vi "Test2_3b.vi"(0 "Instrument VISA in":T1={"AWG VISA"="81160A", "Oscilloscope  VISA "="Oscilloscope", "Integration Board IP"="172.16.7.43", "connection ID"=refnum, "report out"=refnum, "report file path"=path "D:/CTA/Data_test/adds"}, 7 "Cycles Burst":i32=10000, 9 "L1 Address":i32=17, 11 "error in":errorcluster, 12 "channel array":i32[](array[numeric])=[0, 1, 2, 3, 4, 5, 6], 13 "L1 version":bool) -> (4 "Instrument VISA out":T1={"AWG VISA"="81160A", "Oscilloscope  VISA "="Oscilloscope", "Integration Board IP"="172.16.7.43", "connection ID"=refnum, "report out"=refnum, "report file path"=path "D:/CTA/Data_test/adds"}, 15 "error out":errorcluster)   [LabVIEW 2009]
uses:
  <vilib>/Utility/NIReport.llb/NI_report.lvclass
  <instrlib>/Agilent 81150/Agilent 81150.lvlib
  <instrlib>/Agilent 8000 Series/Agilent 8000 Series.lvlib
panel:
  in  "Voltage":dbl[](array[numeric])=[0.05, 0.1, 0.2, 0.3, 0.4, 0.5, 0.6, 0.7, 0.8, 0.9, 1.0, 1.1, 1.2]
  in  "quantity":i32=2
  in  "cliipping":i32[](array[numeric])=[380, 381, 396, 376, 369, 371, 333]
  in  "attenuation":i32[](array[numeric])=[1574, 1572, 1542, 1574, 1569, 1563, 1581]
  out "IPR_Address":i32=23
  out "L1 Address":i32=17
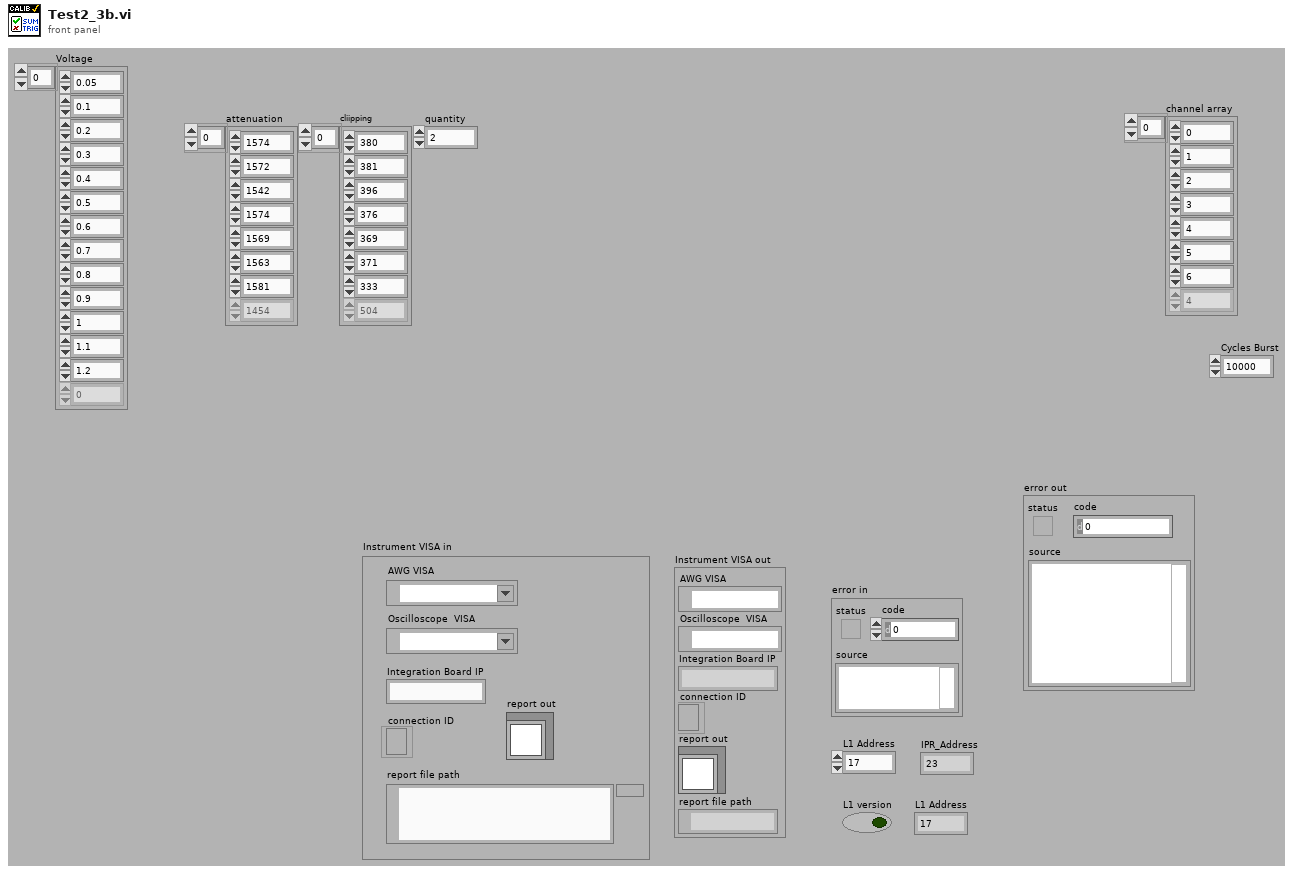
[diagram p1: front panel]
types:
  T1 = cluster{"AWG VISA":refnum<visa-resource-name>, "Oscilloscope  VISA ":refnum<visa-resource-name>, "Integration Board IP":string, "connection ID":refnum<k5>, "report out":refnum<class "NI_report.lvclass">, "report file path":path}
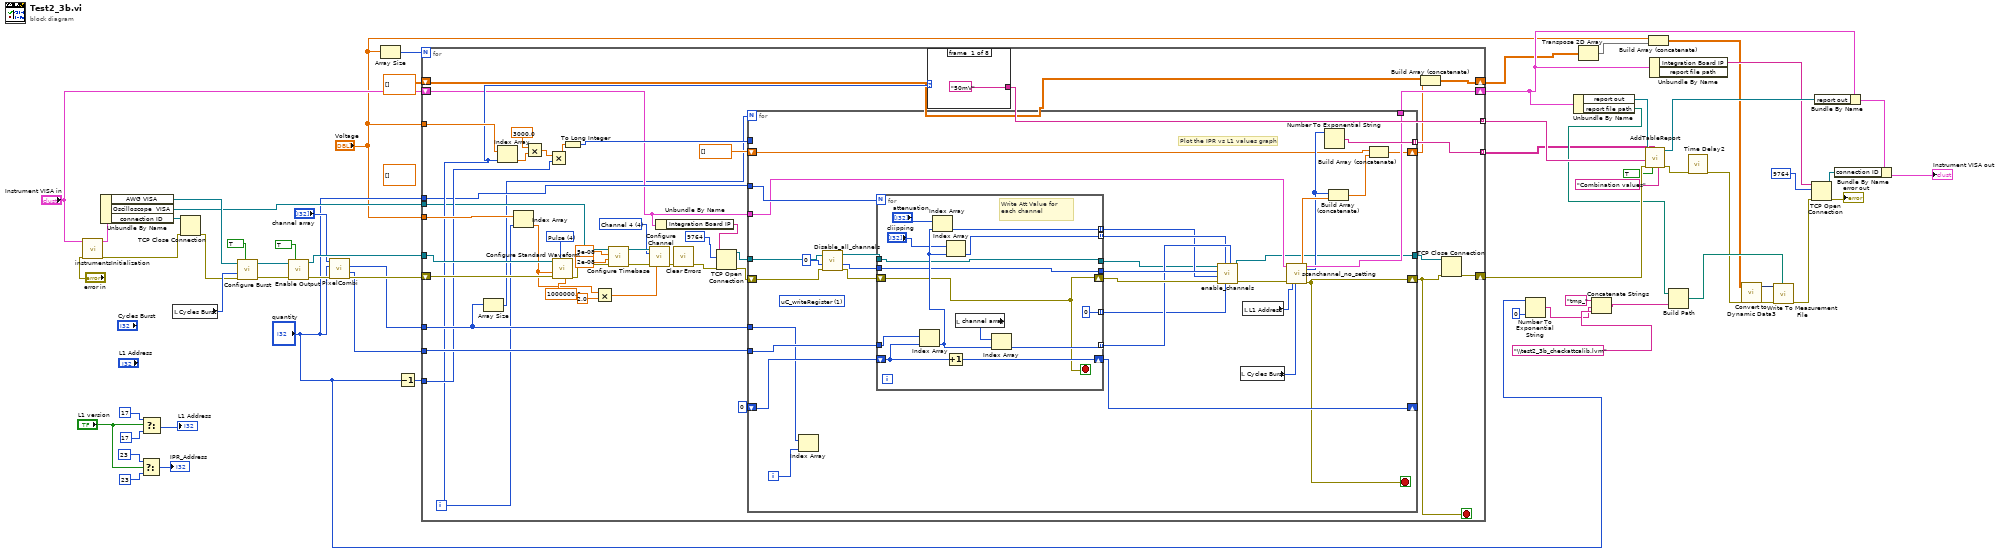
[diagram p0: block diagram]
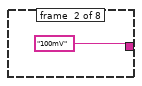
[diagram p2: hidden frame]
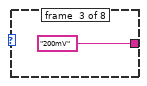
[diagram p3: hidden frame]
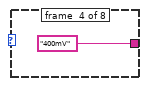
[diagram p4: hidden frame]
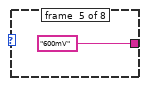
[diagram p5: hidden frame]
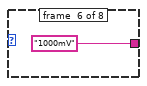
[diagram p6: hidden frame]
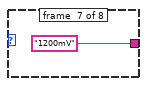
[diagram p7: hidden frame]
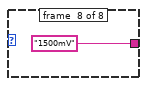
[diagram p8: hidden frame]
diagram:
  (unwired) dbl[][] []
  n1 = call "instrumentsInitialization.vi"("error in"="error in", "Instrument VISA in"="Instrument VISA in") -> ("error out"=w18:errorcluster, "Instrument VISA out"=w20:T1)  [unwired: 8 in]
  n2 = Unbundle By Name(w20) -> ("AWG VISA"=w21:refnum<visa-resource-name>, "Oscilloscope  VISA"=w16:refnum<visa-resource-name>, "connection ID"=w19:refnum<k5>)
  n3 = Select(t=23 ("Address"), s="L1 version", f=23 ("Address")) -> (s? t:f=→"IPR_Address":i32)
  n4 = Select(t=17 ("Address"), s="L1 version", f=17 ("Address")) -> (s? t:f=→"L1 Address":i32)
  n5 = local read "Cycles Burst"() -> (w57:i32)
  n6 = TCP Close Connection(connection ID=w19, error in (no error)=w18) -> (error out=w17:errorcluster)  [unwired: 1 in, 1 out]
  n7 = call <instrlib>:"Configure Burst.vi"("Enable Burst (F: Disable)"=TRUE, "error in (no error)"=w17, "Burst Count (2)"=w57, "VISA resource name"=w21) -> ("error out"=w56:errorcluster, "VISA resource name out"=w55:refnum<visa-resource-name>)  [unwired: 6 in]
  n8 = call <instrlib>:"Enable Output.vi"("Enable Output (T: Enable)"=TRUE, "error in (no error)"=w56, "VISA resource name"=w55) -> ("error out"=w54:errorcluster, "VISA resource name out"=w52:refnum<visa-resource-name>)  [unwired: 7 in]
  n9 = call "PixelCombi.vi"("error in"=w54, "quantity"="quantity", "array"="channel array") -> ("error out"=w53:errorcluster, "Channels"=w51:i32[], "Combination Array"=w50:i16[])  [unwired: 6 in]
  n10 = Array Size(array="Voltage") -> (size(s)=w24:i32)
  n11 = Decrement(x="quantity") -> (x-1=w23:i32)
  n12 = for {
    N: w24 -> [_]
    tunnel: w52 -> [w101]
    tunnel: w51 -> [w100]
    tunnel: w50 -> [w95]
    shift-right: [w60] -> w36
    shift-left: w53 -> [w102]
    tunnel: [w98] -> w7 mode=indexing
    tunnel: [w97] -> w35 mode=indexing
    tunnel: "Voltage" -> [w94]
    tunnel: "Voltage" -> [w93]
    tunnel: w23 -> [w90]
    tunnel: "quantity" -> [w87]
    tunnel: w16 -> [w82]
    shift-right: [w80] -> w14
    shift-left: "Instrument VISA in" -> [w69]
    shift-right: [w73] -> w4
    shift-left: dbl[][] [] -> [w72]
    i -> [w88]
    stop <- w61 stop-if-true
    w77 = 4 items=["Channel 1"=1, "Channel 2"=2, "Channel 3"=3, "Channel 4"=4] ("Channel (1: Channel 1)")
    w104 = u16 4 items=["Sine", "Square", "Ramp Up", "Ramp Down", "Pulse", "Noise", "DC"] ("Waveform (0: Sine)")
    n13 = Array Size(array=w95) -> (size(s)=w63:i32)
    n14 = Index Array(array=w93, index=w88) -> (element=w91:dbl)
    n15 = Index Array(array=w94, index=w88) -> (element=w75:dbl)
    n16 = Multiply(x=3000.0, y=w91) -> (x*y=w89:dbl)
    n17 = Multiply(x=w89, y=w90) -> (x*y=w86:dbl)
    n18 = call <instrlib>:"Configure Standard Waveform.vi"("Frequency (1000.0 Hz)"=1000000.0, "Waveform (0: Sine)"=w104, "error in (no error)"=w102, "Amplitude (1.0 Vpp)"=w75, "VISA resource name"=w101) -> ("error out"=w85:errorcluster)  [unwired: 5 in, 1 out]
    n19 = To Long Integer(number=w86) -> (32bit integer=w99:i32)
    n20 = Multiply(x=w75, y=2.0) -> (x*y=w76:dbl)
    n21 = call <instrlib>:"Configure Timebase.vi"("error in (no error)"=w85, "Position (0.0 s)"=2e-08, "Timebase (0.005 s)"=5e-08, "VISA resource name"=w82) -> ("error out"=w84:errorcluster, "VISA resource name out"=w81:refnum<visa-resource-name>)  [unwired: 6 in]
    n22 = call <instrlib>:"Configure Channel.vi"("VISA resource name"=w81, "Channel (1: Channel 1)"=w77, "error in (no error)"=w84, "Vertical Range (2.0 V)"=w76) -> ("error out"=w83:errorcluster)  [unwired: 10 in, 1 out]
    n23 = Unbundle By Name(w69) -> ("Integration Board IP"=w66:string)
    n24 = call <vilib>:"Clear Errors.vi"("error in (no error)"=w83) -> ("error out"=w68:errorcluster)  [unwired: 6 in]
    n25 = TCP Open Connection(address=w66, remote port or service name=u16 9764, error in (no error)=w68) -> (connection ID=w64:refnum<k5>, error out=w67:errorcluster)  [unwired: 2 in]
    n26 = for {
      N: w63 -> [_]
      tunnel: w95 -> [w141]
      tunnel: w100 -> [w142]
      shift-right: [w143] -> _
      shift-left: i16 0 ("element") -> [w144]
      shift-right: [w125] -> w61
      shift-left: w67 -> [w115]
      tunnel: w69 -> [w123]
      tunnel: w87 -> [w140]
      tunnel: w99 -> [_]
      tunnel: [w139] -> w98 mode=indexing
      tunnel: [w122] -> w80
      shift-right: [w117] -> w70
      shift-left: dbl[] [] ("element") -> [w119]
      tunnel: w64 -> [w116]
      tunnel: [w114] -> w62
      i -> [w138]
      stop <- w125 stop-if-true
      (unwired) u16 1 items=["sendCommand"=9, "FPGA_writeRegister"=3, "FPGA_readRegister"=2, "uC_writeRegister"=1, "uC_readRegister"=0] ("Action")
      # "Plot the IPR vs L1 values graph"
      n27 = Index Array(array=w141, index=w138) -> ()  [unwired: 1 out]
      n28 = call "Disable_all_channels.vi"("error in"=w115, "id_in"=0 ("Data"), "connection ID"=w116) -> ("error out"=w136:errorcluster, "id_out"=w132:i32, "connection ID out"=w135:refnum<k5>)  [unwired: 6 in]
      n29 = for {
        N: w140 -> [_]
        shift-right: [w157] -> w143
        shift-left: w144 -> [w158]
        tunnel: w142 -> [w156]
        tunnel: [w147] -> w128
        shift-right: [w146] -> w134
        shift-left: w136 -> [w146]
        tunnel: w135 -> [w147]
        tunnel: [w151] -> w133
        tunnel: w132 -> [w151]
        tunnel: [w150] -> w131 mode=indexing
        tunnel: [w149] -> w130 mode=indexing
        tunnel: [w148] -> w129 mode=indexing
        tunnel: [0 ("State machine")] -> w127 mode=indexing
        stop <- w146 stop-if-true
        # "Write Att Value for each channel"
        n30 = Index Array(array=w156, index=w158) -> (element=w153:i32)
        n31 = Index Array(array="attenuation", index=w153) -> (element=w148:i32)
        n32 = Index Array(array="cliipping", index=w153) -> (element=w149:i32)
        n33 = Increment(x=w158) -> (x+1=w157:i16)
        n34 = local read "channel array"() -> (w155:i32[])
        n35 = Index Array(array=w155, index=w153) -> (element=w150:i32)
      }
      n36 = call "enable_channels.vi"("channel"=w131, "celay"=w127, "vclip"=w130, "error in"=w134, "vatt"=w129, "id_in"=w133, "connection ID"=w128) -> ("error out"=w113:errorcluster, "connection ID out"=w114:refnum<k5>)  [unwired: 2 in, 1 out]
      n37 = local read "Cycles Burst"() -> (w126:i32)
      n38 = local read "L1 Address"() -> (w124:i32)
      n39 = call "scanchannel_no_setting.vi"("Instrument VISA in"=w123, "error in"=w113, "L1 Address"=w124, "Ch burst"=w126) -> ("appended array"=w121:dbl[], "output cluster"=w122:T1, "L1 value"=w120:i32, "error out"=w125:errorcluster)  [unwired: 10 in, 2 out]
      n40 = Number To Exponential String(number=w120) -> (E-format string=w139:string)  [unwired: 3 in]
      n41 = Build Array (concatenate)(w120, w121) -> (w118:dbl[])
      n42 = Build Array (concatenate)(w119, w118) -> (w117:dbl[])
    }
    n43 = case shown="0, Default" w88 {
      tunnel: ["50mV" ("regular expression") "100mV" ("regular expression") "200mV" ("regular expression") "400mV" ("regular expression") "600mV" ("regular expression") "1000mV" ("regular expression") "1200mV" ("regular expression") "1500mV" ("regular expression")] -> w97
      frame #0 {
      }
      frame #1 {
      }
      frame #2 {
      }
      frame #3 {
      }
      frame #4 {
      }
      frame #5 {
      }
      frame #6 {
      }
      frame #7 {
      }
    }
    n44 = Build Array (concatenate)(w72, w70) -> (w73:dbl[][])
    n45 = TCP Close Connection(connection ID=w62, error in (no error)=w61) -> (error out=w60:errorcluster)  [unwired: 1 in, 1 out]
  }
  n46 = Number To Exponential String(number="quantity", precision (6)=i16 0) -> (E-format string=w9:string)  [unwired: 2 in]
  n47 = Unbundle By Name(w14) -> ("report out"=w39:refnum<class "NI_report.lvclass">, "report file path"=w28:path)
  n48 = Transpose 2D Array(2D array=w4) -> (transposed array=w3:dbl[][])
  n49 = Concatenate Strings("tmp_" ("string"), w9, "\\test2_3b_checkattcalib.lvm" ("name or relative path")) -> (w12:string)
  n50 = call "AddTableReport.vi"("Table title"="Combination values", "Report Enable"=TRUE, "Data"=w7, "error in"=w36, "Columns"=w35, "report in"=w39) -> ("error out"=w32:errorcluster, "report out"=w37:refnum<class "NI_report.lvclass">)  [unwired: 4 in]
  n51 = Build Array (concatenate)("Voltage", w3) -> (w2:dbl[][])
  n52 = Unbundle By Name(w14) -> ("Integration Board IP"=w13:string)  [unwired: 1 out]
  n53 = Build Path(base path=w28, name or relative path=w12) -> (appended path=w27:path)
  n54 = call "Time Delay2"("error in (no error)"=w32) -> ("error out"=w25:errorcluster)  [unwired: 10 in]
  n55 = call "Convert to Dynamic Data3"("2D Array"=w2) -> ("Dynamic Data Type"=w29:dynamicdata)  [unwired: 3 in]
  n56 = call "Write To Measurement File"("Signals"=w29, "error in (no error)"=w25, "Filename"=w27) -> ("error out"=w26:errorcluster)  [unwired: 14 in, 2 out]
  n57 = TCP Open Connection(address=w13, remote port or service name=u16 9764, error in (no error)=w26) -> (connection ID=w48:refnum<k5>, error out=→"error out":errorcluster)  [unwired: 2 in]
  n58 = Bundle By Name(cluster=w14, "report out"=w37) -> (w38:T1)
  n59 = Bundle By Name(cluster=w38, "connection ID"=w48) -> (→"Instrument VISA out":T1)
